vi "Add wprot init.vi"(8 "error in (no error)":errorcluster, 11 "ICS in":refnum<class "ICS.lvclass">) -> (0 "error out":errorcluster, 3 "ICS out":refnum<class "ICS.lvclass">)   [LabVIEW 2018, in "ICS.lvclass"]
uses:
  ICS.lvclass
  ICS.lvclass/ICS.ctl
  Motor/Motor.lvclass
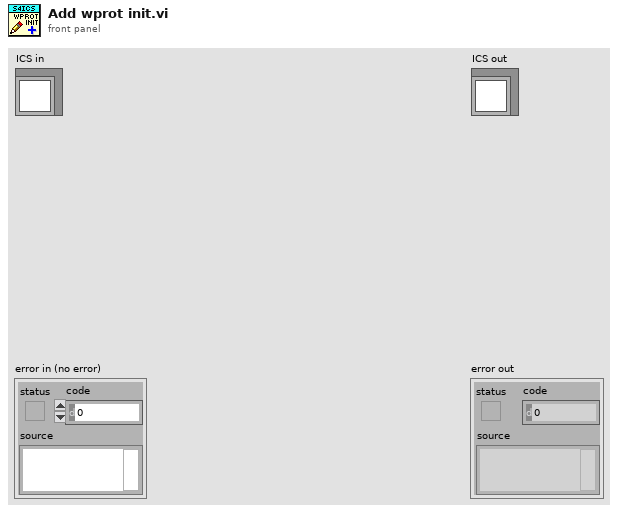
[diagram p1: front panel]
types:
  T1 = cluster{"action":string, "param":string, "pos_name":string, "pos_idx":i32, "ack":bool, "stop":bool, "offset":bool, "immediate":bool, "instructions":string[]}
  T2 = cluster{"mode":string, "condition":string, "position":string, "pos_name":string, "pos_id":string}
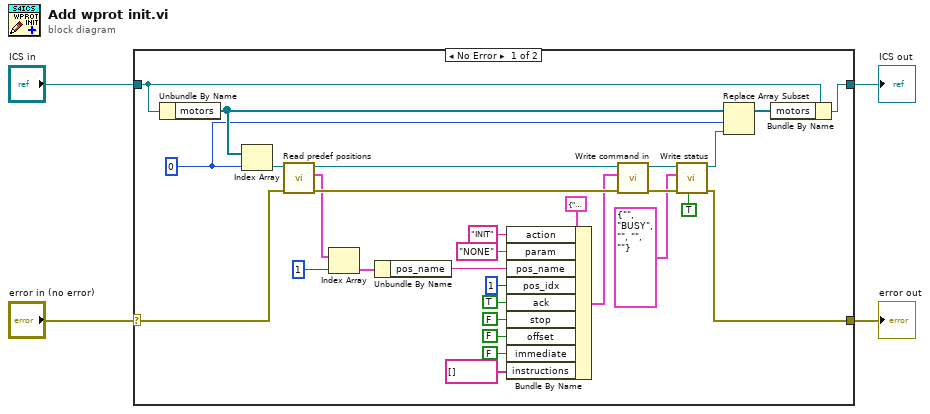
[diagram p0: block diagram]
diagram:
  n1 = case shown="No Error" "error in (no error)" {
    selector: "error in (no error)" -> [w22 w34]
    tunnel: [w25 w34] -> w3
    tunnel: [w33 w35] -> w1
    tunnel: "ICS in" -> [w32 w35]
    frame No Error {
      w29 = 0 ("index")
      n2 = Unbundle By Name(w32) -> ("motors"=w30:refnum<class "Motor.lvclass">[])
      n3 = Index Array(array=w30, index=w29) -> (element=w21:refnum<class "Motor.lvclass">)
      n4 = call-dynamic "Read predef positions.vi"("error in (no error)"=w22, "Motor in"=w21) -> ("error out"=w19:errorcluster, "predef positions"=w18:cluster{"pos_name":string, "pos_value":dbl}[], "Motor out"=w20:refnum<class "Motor.lvclass">)  [unwired: 7 in]
      n5 = Index Array(array=w18, index=1) -> (element=w16:cluster{"pos_name":string, "pos_value":dbl})
      n6 = Unbundle By Name(w16) -> ("pos_name"=w15:string)
      n7 = Bundle By Name(cluster=T1 {"action"="", "param"="", "pos_name"="", "pos_idx"=0, "ack"=FALSE, "stop"=FALSE, "offset"=FALSE, "immediate"=FALSE, "instructions"=[]} ("command in"), "action"="INIT", "param"="NONE", "pos_name"=w15, "pos_idx"=1, "ack"=TRUE, "stop"=FALSE, "offset"=FALSE, "immediate"=FALSE, "instructions"=string[] []) -> (w7:T1)
      n8 = call-dynamic "Write command in.vi"("error in (no error)"=w19, "command in"=w7, "Motor in"=w20) -> ("error out"=w26:errorcluster, "Motor out"=w28:refnum<class "Motor.lvclass">)  [unwired: 7 in]
      n9 = call-dynamic "Write status.vi"("hold if empty"=TRUE, "error in (no error)"=w26, "status"=T2 {"mode"="", "condition"="BUSY", "position"="", "pos_name"="", "pos_id"=""}, "Motor in"=w28) -> ("error out"=w25:errorcluster, "Motor out"=w27:refnum<class "Motor.lvclass">)  [unwired: 6 in]
      n10 = Replace Array Subset(array=w30, new element=w27, index=w29) -> (w31:refnum<class "Motor.lvclass">[])
      n11 = Bundle By Name(cluster=w32, "motors"=w31) -> (w33:refnum<class "ICS.lvclass">)
    }
    frame Error {
    }
  }
  "error out" <- w3
  "ICS out" <- w1
